vi "Color_Project.vi"() -> ()   [LabVIEW 2014]
uses:
  leitura de dados txt control.ctl
panel:
  out "Chromaticity diagram":cluster{dbl, dbl}[](graph)
  out "Selected illuminant":dbl[](array[numeric])
  out "Z":dbl
  out "Y":dbl
  out "X":dbl
  out "Reflectance":i32[](array[numeric])
  out "Is CMF selected?":bool
  out "Is illuminant selected?":bool
  out "Intepoled iluminants":dbl[][](array[numeric])
  out "Selected\nCMF":dbl[][](array[numeric])
  out "cmf Index":dbl
  out "CMFCols":i32
  out "CMFRows":i32
  out "CMF Table":string[][](array[string])
  in  "Color Matching Function":string(combo)
  out "ILCols":i32
  out "ILRows":i32
  out "Illuminant Graph":T1(graph)
  out "GammaInterval":dbl[](array[numeric])
  out "NeedInterpolation?":bool
  out "Illuminant Tabel":string[][](array[string])
  out "Selected illuminant index":dbl
  in  "Select Illuminant":T2
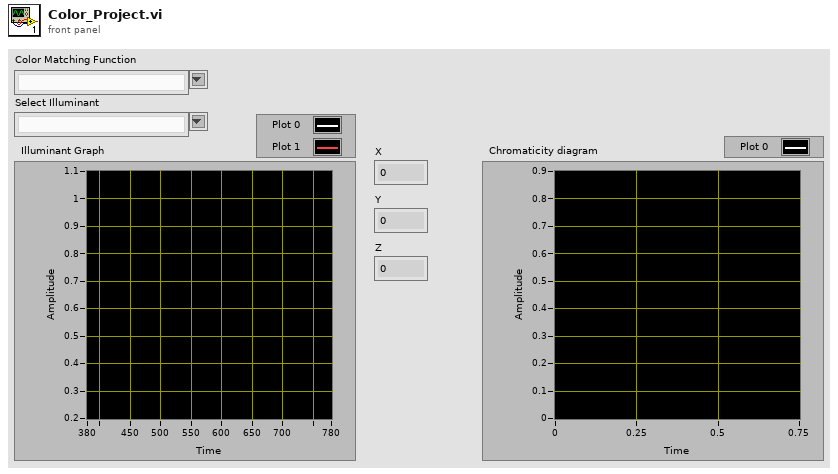
[diagram p1: front panel]
types:
  T1 = cluster{"GammaInterval":dbl[], "Interpolated":dbl[]}[]
  T2 = typedef "leitura de dados txt control.ctl" = string
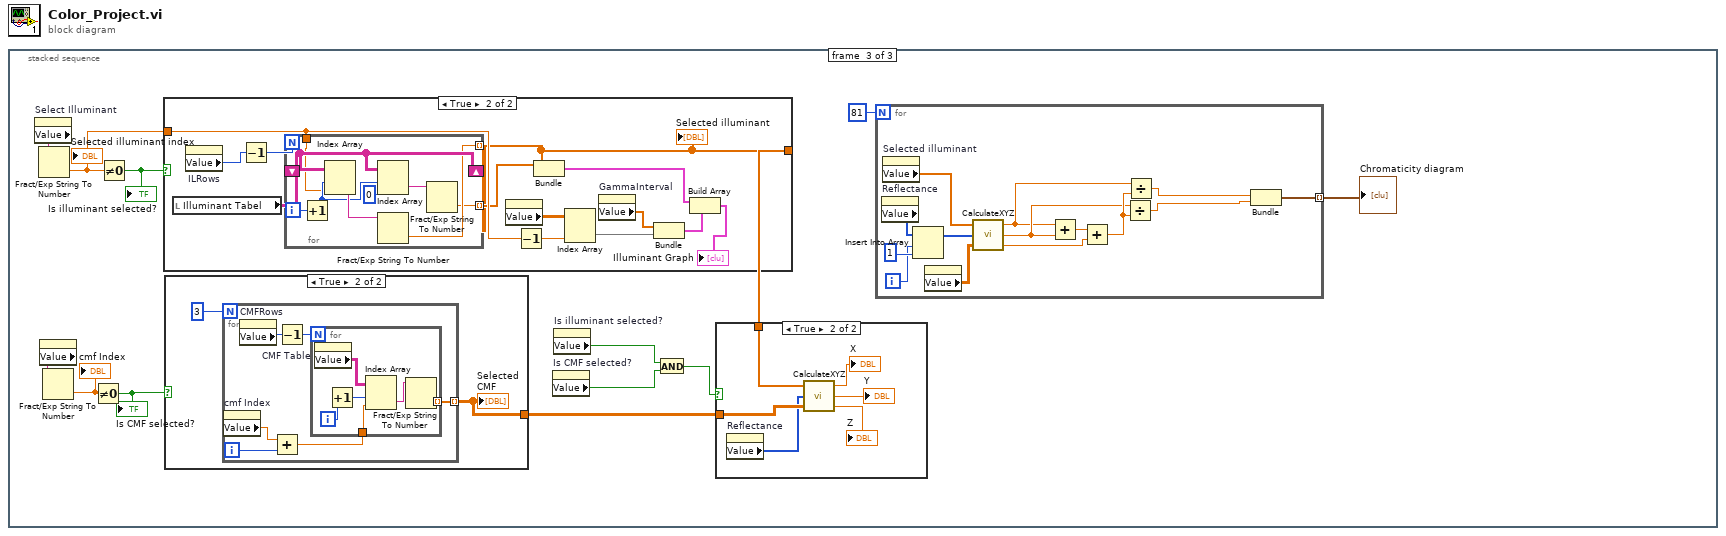
[diagram p0: block diagram]
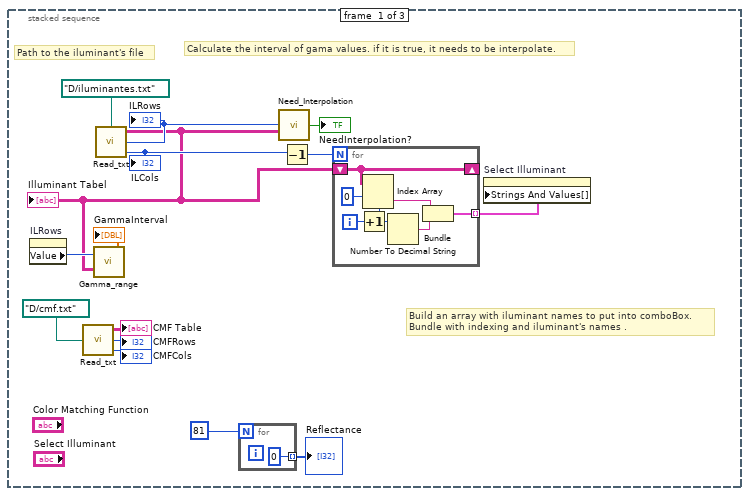
[diagram p2: hidden frame]
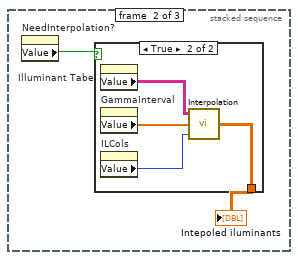
[diagram p3: hidden frame]
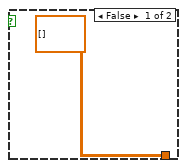
[diagram p4: hidden frame]
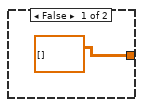
[diagram p6: hidden frame]
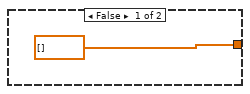
[diagram p7: hidden frame]
diagram:
  n1 = stacked-sequence {
    frame #0 {
      # "Calculate the interval of gama values. if it is true, it needs to be interpolate."
      # "Path to the iluminant's file"
      # "Build an array with iluminant names to put into comboBox.\nBundle with indexing and iluminant's names ."
      n2 = property on="ILRows" class="DigNum (strict)"() -> ("Value"=w8:i32)  [unwired: 2 in, 2 out]
      n3 = call "Read_txt.vi"("file path (dialog if empty)"=path "D:/cmf.txt") -> ("Elements"=→"CMF Table":string[][], "Rows"=→"CMFRows":i32, "Cols"=→"CMFCols":i32)
      n4 = call "Read_txt.vi"("file path (dialog if empty)"=path "D:/iluminantes.txt") -> ("Elements"=w7:string[][], "Rows"=w11:i32, "Cols"=w10:i32)
      "Illuminant Tabel" <- w7
      "ILRows" <- w11
      "ILCols" <- w10
      n5 = call "Gamma_range.vi"("Illuminant Table"=w7, "NumberOfRows"=w8) -> ("GammaInterval"=→"GammaInterval":dbl[])
      n6 = for {
        N: 81 -> [_]
        tunnel: [0] -> w1 mode=indexing
      }
      "Reflectance" <- w1
      n7 = call "Need_Interpolation.vi"("Matrix with txt"=w7, "Number of Rows"=w11) -> ("isNotFive?"=→"NeedInterpolation?":bool)
      n8 = Decrement(x=w10) -> (x-1=w14:i32)
      n9 = for {
        N: w14 -> [_]
        shift-right: [w21] -> _
        shift-left: w7 -> [w21]
        tunnel: [w17] -> w15 mode=indexing
        i -> [w23]
        n10 = Increment(x=w23) -> (x+1=w20:i32)
        n11 = Index Array(array=w21, index (row)=0, index (col)=w20) -> (element=w18:string)
        n12 = Number To Decimal String(number=w20) -> (decimal integer string=w19:string)  [unwired: 1 in]
        n13 = Bundle("String"=w18, w19) -> (w17:cluster{"String":string, string})  [unwired: 1 in]
      }
      n14 = property on="Select Illuminant" class="CmbBox (strict)"("Strings And Values[]"=w15) -> ()  [unwired: 2 in, 2 out]
    }
    frame #1 {
      n15 = property on="NeedInterpolation?" class="Bool (strict)"() -> ("Value"=w25:bool)  [unwired: 2 in, 2 out]
      n16 = case shown="True" w25 {
        tunnel: [dbl[][] [] w27] -> w24
        frame False {
        }
        frame True {
          n17 = property on="Illuminant Tabel" class="Arr (strict)"() -> ("Value"=w30:string[][])  [unwired: 2 in, 2 out]
          n18 = property on="GammaInterval" class="Arr (strict)"() -> ("Value"=w29:dbl[])  [unwired: 2 in, 2 out]
          n19 = property on="ILCols" class="DigNum (strict)"() -> ("Value"=w28:i32)  [unwired: 2 in, 2 out]
          n20 = call "Interpolation.vi"("Number of Columns"=w28, "Lambda Interval"=w29, "Illuminants"=w30) -> ("Interpolated"=w27:dbl[][])
        }
      }
      "Intepoled iluminants" <- w24
    }
    frame #2 {
      n21 = property on="Select Illuminant" class="CmbBox (strict)"() -> ("Value"=w39:T2)  [unwired: 2 in, 2 out]
      n22 = Fract/Exp String To Number(string=w39) -> (number=w38:dbl)  [unwired: 3 in, 1 out]
      "Selected illuminant index" <- w38
      n23 = property on="Color Matching Function" class="CmbBox"() -> ("Value"=w41:string)  [unwired: 2 in, 2 out]
      n24 = Fract/Exp String To Number(string=w41) -> (number=w42:dbl)  [unwired: 3 in, 1 out]
      "cmf Index" <- w42
      n25 = Not Equal To 0?(x=w42) -> (x != 0?=w40:bool)
      "Is CMF selected?" <- w40
      n26 = Not Equal To 0?(x=w38) -> (x != 0?=w43:bool)
      "Is illuminant selected?" <- w43
      n27 = case shown="True" w43 {
        tunnel: w38 -> [_ w87]
        tunnel: [dbl[] [] w80] -> w32
        frame False {
        }
        frame True {
          n28 = local read "Illuminant Tabel"() -> (w91:string[][])
          n29 = property on="ILRows" class="DigNum (strict)"() -> ("Value"=w85:i32)  [unwired: 2 in, 2 out]
          n30 = Decrement(x=w85) -> (x-1=w92:i32)
          n31 = for {
            N: w92 -> [_]
            shift-right: [w100] -> _
            shift-left: w91 -> [w100]
            tunnel: w87 -> [w93]
            tunnel: [w95] -> w80 mode=indexing
            tunnel: [w94] -> w82 mode=indexing
            i -> [w101]
            n32 = Increment(x=w101) -> (x+1=w96:i32)
            n33 = Index Array(array=w100, index (row)=w96, index (col)=w93) -> (element=w97:string)
            n34 = Index Array(array=w100, index (row)=w96, index (col)=0 ("disabled index (col)")) -> (element=w98:string)
            n35 = Fract/Exp String To Number(string=w97) -> (number=w95:dbl)  [unwired: 3 in, 1 out]
            n36 = Fract/Exp String To Number(string=w98) -> (number=w94:dbl)  [unwired: 3 in, 1 out]
          }
          "Selected illuminant" <- w80
          n37 = property on="Intepoled iluminants" class="Arr (strict)"() -> ("Value"=w84:dbl[][])  [unwired: 2 in, 2 out]
          n38 = Decrement(x=w87) -> (x-1=w86:dbl)
          n39 = Bundle(w82, w80) -> (w88:cluster{dbl[], dbl[]})  [unwired: 1 in]
          n40 = Index Array(array=w84, index (col)=w86) -> (element=w81:dbl[])  [unwired: 1 in]
          n41 = property on="GammaInterval" class="Arr (strict)"() -> ("Value"=w83:dbl[])  [unwired: 2 in, 2 out]
          n42 = Bundle("Value"=w83, "Value"=w81) -> (w89:cluster{"Value":dbl[], "Value":dbl[]})  [unwired: 1 in]
          n43 = Build Array(w88, w89) -> (→"Illuminant Graph":cluster{"Value":dbl[], "Value":dbl[]}[])
        }
      }
      n44 = case shown="True" w40 {
        tunnel: [dbl[][] [] w65] -> w34
        frame False {
        }
        frame True {
          n45 = for {
            N: 3 -> [_]
            tunnel: [w69] -> w65 mode=indexing
            i -> [w71]
            n46 = property on="cmf Index" class="DigNum (strict)"() -> ("Value"=w72:dbl)  [unwired: 2 in, 2 out]
            n47 = property on="CMFRows" class="DigNum (strict)"() -> ("Value"=w68:i32)  [unwired: 2 in, 2 out]
            n48 = Add(x=w72, y=w71) -> (x+y=w70:dbl)
            n49 = Decrement(x=w68) -> (x-1=w67:i32)
            n50 = for {
              N: w67 -> [_]
              tunnel: w70 -> [w77]
              tunnel: [w73] -> w69 mode=indexing
              i -> [w76]
              n51 = property on="CMF Table" class="Arr (strict)"() -> ("Value"=w78:string[][])  [unwired: 2 in, 2 out]
              n52 = Increment(x=w76) -> (x+1=w75:i32)
              n53 = Index Array(array=w78, index (row)=w75, index (col)=w77) -> (element=w74:string)
              n54 = Fract/Exp String To Number(string=w74) -> (number=w73:dbl)  [unwired: 3 in, 1 out]
            }
          }
          "Selected\nCMF" <- w65
        }
      }
      n55 = property on="Is CMF selected?" class="Bool (strict)"() -> ("Value"=w36:bool)  [unwired: 2 in, 2 out]
      n56 = property on="Is illuminant selected?" class="Bool (strict)"() -> ("Value"=w37:bool)  [unwired: 2 in, 2 out]
      n57 = And(x=w37, y=w36) -> (x .and. y?=w35:bool)
      n58 = case shown="True" w35 {
        tunnel: w32 -> [_ w63]
        tunnel: w34 -> [_ w62]
        frame False {
        }
        frame True {
          n59 = property on="Reflectance" class="Arr (strict)"() -> ("Value"=w61:i32[])  [unwired: 2 in, 2 out]
          n60 = call "CalculateXYZ.vi"("CMF"=w62, "Reflectance"=w61, "Illuminant"=w63) -> ("Z"=→"Z":dbl, "Y"=→"Y":dbl, "X"=→"X":dbl)
        }
      }
      n61 = for {
        N: 81 -> [_]
        tunnel: [w47] -> w31 mode=indexing
        i -> [w50]
        n62 = property on="Reflectance" class="Arr (strict)"() -> ("Value"=w56:i32[])  [unwired: 2 in, 2 out]
        n63 = property on="Selected illuminant" class="Arr (strict)"() -> ("Value"=w53:dbl[])  [unwired: 2 in, 2 out]
        n64 = Insert Into Array(array=w56, index=w50, new element=1 ("new element/subarray")) -> (w54:i32[])
        n65 = property on="Selected\nCMF" class="Arr (strict)"() -> ("Value"=w55:dbl[][])  [unwired: 2 in, 2 out]
        n66 = call "CalculateXYZ.vi"("CMF"=w55, "Reflectance"=w54, "Illuminant"=w53) -> ("Z"=w46:dbl, "Y"=w45:dbl, "X"=w44:dbl)
        n67 = Add(x=w44, y=w45) -> (x+y=w52:dbl)
        n68 = Add(x=w52, y=w46) -> (x+y=w51:dbl)
        n69 = Divide(x=w45, y=w51) -> (x/y=w48:dbl)
        n70 = Divide(x=w44, y=w51) -> (x/y=w49:dbl)
        n71 = Bundle(w49, w48) -> (w47:cluster{dbl, dbl})  [unwired: 1 in]
      }
      "Chromaticity diagram" <- w31
    }
  }
